vi "KH_DAQ_FGlob_AO.vi"(5 "Function (Recall One)":T1=enum."Recall one", 6 "Alarm":bool, 7 "PXI AO_Item":u16, 8 "err in":errorcluster caption="error", 10 "AO Values IN":sgl[](array[numeric]) format="%.6f", 11 "AO Value IN":sgl format="%.6f") -> (0 "err out":errorcluster caption="error", 2 "AO Values OUT":sgl[](array[numeric]) format="%.6f", 3 "AO Value OUT":sgl format="%.6f")   [LabVIEW 2021]
uses:
  KH Turck EthernetIP 17.12/KH TURCK TypeDefs FGlob.ctl
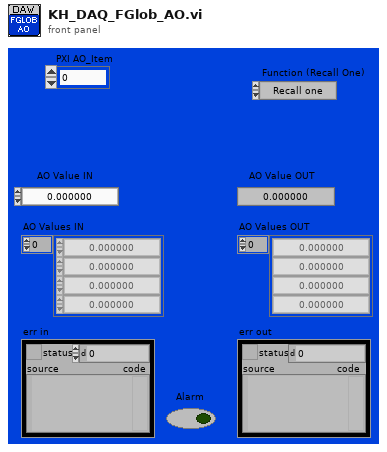
[diagram p1: front panel]
types:
  T1 = typedef "KH TURCK TypeDefs FGlob.ctl" = enum16{"Put one", "Put all", "Recall one", "Recall all"}
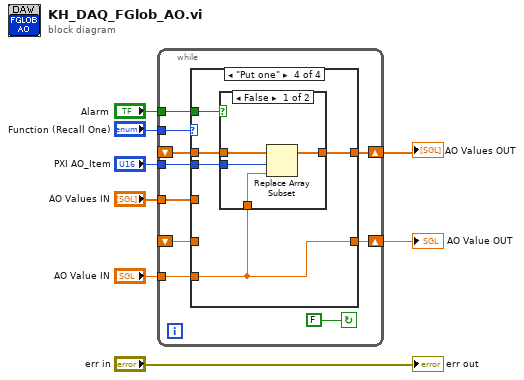
[diagram p0: block diagram]
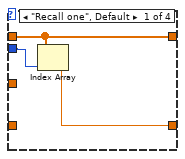
[diagram p2: hidden frame]
diagram:
  n1 = while {
    shift-right: [w16] -> w6
    shift-left: _ -> [w15]
    tunnel: "Function (Recall One)" -> [w17]
    tunnel: "PXI AO_Item" -> [w13]
    tunnel: "AO Values IN" -> [w12]
    shift-right: [w14] -> w5
    shift-left: _ -> [w11]
    tunnel: "AO Value IN" -> [w10]
    tunnel: "Alarm" -> [w9]
    stop <- FALSE continue-if-true
    n2 = case shown="\"Put one\"" w17 {
      tunnel: [w21 w23 w24 w34] -> w16
      tunnel: w15 -> [w21 w23 w25 w35]
      tunnel: w13 -> [w20 _ _ w33]
      tunnel: [w19 w22 w28 w32] -> w14
      tunnel: w12 -> [_ _ w27 _]
      tunnel: w11 -> [_ w22 w28 _]
      tunnel: w10 -> [_ _ _ w32]
      tunnel: w9 -> [_ _ w26 w31]
      frame "Recall one", Default {
        n3 = Index Array(array=w21, index=w20) -> (element=w19:sgl)
      }
      frame "Recall all" {
      }
      frame "Put all" {
        n4 = case shown="False" w26 {
          tunnel: w27 -> [w29 _]
          tunnel: w25 -> [_ w30]
          tunnel: [w29 w30] -> w24
          frame False {
          }
          frame True {
          }
        }
      }
      frame "Put one" {
        n5 = case shown="False" w31 {
          tunnel: w35 -> [w39 w40]
          tunnel: [w38 w40] -> w34
          tunnel: w33 -> [w37 _]
          tunnel: w32 -> [w36 _]
          frame False {
            n6 = Replace Array Subset(array=w39, new element=w36, index=w37) -> (w38:sgl[])
          }
          frame True {
          }
        }
      }
    }
  }
  "AO Values OUT" <- w6
  "AO Value OUT" <- w5
  "err out" <- "err in"
